vi "resources read.vi"(8 "error in":errorcluster, 10 "id":i32, 11 "message json":string) -> (0 "error out":errorcluster, 3 "response":string)   [LabVIEW 2025, in "MCP Server.lvlib"]
uses:
  MCP Server.lvlib
  53053a3e-d98d-4b1b-9ea2-8aa51a7e4ea3.vi
  26a76da7-6ace-4620-8e47-f7e66d57a6fb.vi
  a3b2ea05-9a55-4a6d-83fc-f98ed783a032.vi
  e0fbd291-d89e-42a3-8ed1-33df253c9476.vi
  fa2b7325-da3b-4faf-97be-a89ba966e5b3.vi
  <vilib>/JDP Science/JSONtext/Find Item.vi
  <vilib>/JDP Science/JSONtext/Next JSON Value.vi
  <vilib>/JDP Science/JSONtext/String Subset.vi
  <vilib>/JDP Science/JSONtext/Parsing/Advance past next JSON Value (inlined COPY).vi
  <vilib>/JDP Science/JSONtext/Parsing/Advance past whitespace.vi
  <vilib>/JDP Science/JSONtext/Parsing/Advance past String.vi
  <vilib>/JDP Science/JSONtext/Parsing/Advance past Number.vi
  <vilib>/JDP Science/JSONtext/Parsing/Advance past Line Ending.vi
  <vilib>/JDP Science/JSONtext/Parsing/Parse Full Path or Item Name.vi
  <vilib>/JDP Science/JSONtext/Parsing/Advance past Array.vi
  <vilib>/JDP Science/JSONtext/Parsing/Advance past Object.vi
  <vilib>/JDP Science/JSONtext/support/Error Cluster From Code.vi
  <vilib>/JDP Science/JSONtext/Offset/Find Item Locations by Path.vi
  <vilib>/JDP Science/JSONtext/JSON text to Variant.vi
  <vilib>/Utility/error.llb/Error Cluster From Error Code.vi
  <vilib>/JDP Science/JSONtext/Variant to JSON Text.vi
  <vilib>/JDP Science/JSONtext/support/Format JSON Array Text.vi
  <vilib>/JDP Science/JSONtext/support/Format JSON Object.vi
  <vilib>/JDP Science/JSONtext/LVClass Serializer/JSONtext LVClass Serializer.lvclass
  <vilib>/ErrorRing/Error Ring.xnode
  <vilib>/JDP Science/JSONtext/JSONtext.lvlib
  <vilib>/JDP Science/JDP Science Common Utilities/Base64/Base64 Support.lvlib
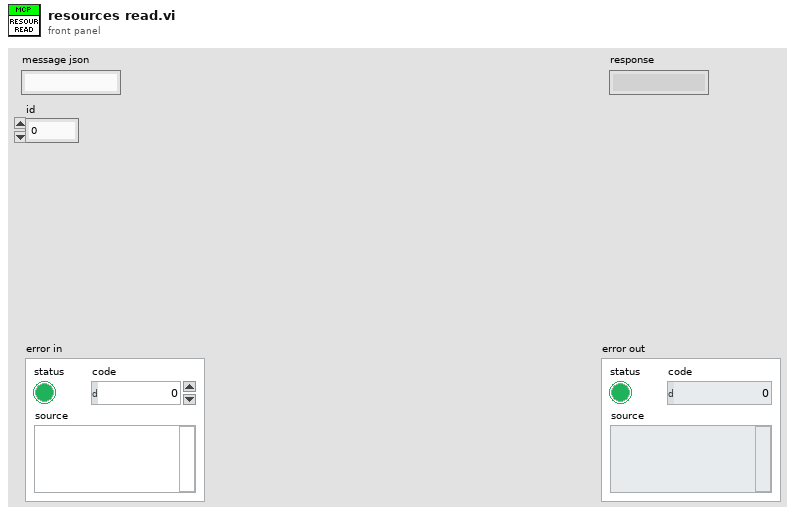
[diagram p1: front panel]
types:
  T1 = typedef "MCP Server.lvlib/resource data.ctl" = cluster{"uri":string, "name":string, "description":string, "mimeType":string, "file path":path}
  T2 = cluster{"uri":string, "mimeType":string, "text":string}
  T3 = cluster{"uri":string, "mimeType":string, "blob":string}
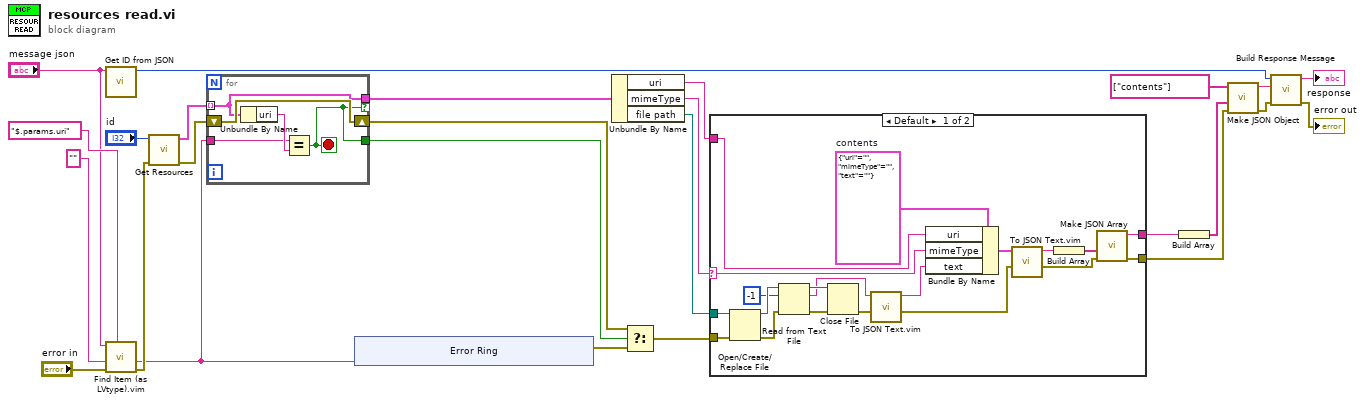
[diagram p0: block diagram]
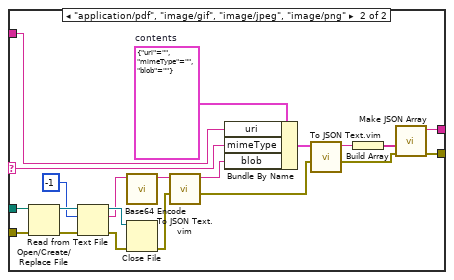
[diagram p2: hidden frame]
diagram:
  n1 = call "Get ID from JSON.vi"("message json"="message json") -> ("Data out"=w8:i32)  [unwired: 10 in]
  n2 = call "Find Item (as LVtype).vim"("$Path or Item Name"="$.params.uri", "error in (no error)"="error in", "Data Type and Default Value"="" ("JSON"), "JSON"="message json") -> ("error out"=w21:errorcluster, "Data"=w12:string)  [unwired: 4 in, 2 out]
  n3 = call "Get Resources.vi"("error in (no error)"=w21, "id"="id") -> ("error out"=w25:errorcluster, "resources"=w22:T1[])  [unwired: 8 in]
  n4 = for {
    shift-right: [w31] -> w23
    shift-left: w25 -> [w31]
    tunnel: w22 -> [w28] mode=indexing
    tunnel: w12 -> [w29]
    tunnel: [w28] -> w18 if=w27
    tunnel: [w27] -> w15
    stop <- w27 stop-if-true
    n5 = Unbundle By Name(w28) -> ("uri"=w30:string)
    n6 = Equal?(x=w29, y=w30) -> (x = y?=w27:bool)
  }
  n7 = xnode "Error Ring"("parameter 0"=w12) -> ("error out"=w16:errorcluster)
  n8 = Unbundle By Name(w18) -> ("uri"=w7:string, "mimeType"=w13:string, "file path"=w6:path)
  n9 = Select(t=w23, s=w15, f=w16) -> (s? t:f=w17:errorcluster)
  n10 = case shown="Default" w13 {
    selector: w13 -> [w44 w65]
    tunnel: w17 -> [w51 w72]
    tunnel: [w37 w59] -> w14
    tunnel: w7 -> [w43 w64]
    tunnel: [w36 w58] -> w3
    tunnel: w6 -> [w33 w55]
    frame Default {
      w45 = T2 {"uri"="", "mimeType"="", "text"=""}  # contents
      n11 = Open/Create/Replace File(file path (use dialog)=w33, error in=w51) -> (refnum out=w47:refnum<file>, error out=w50:errorcluster)  [unwired: 4 in, 1 out]
      n12 = Read from Text File(file (use dialog)=w47, count=-1, error in=w50) -> (refnum out=w46:refnum<file>, text=w41:string, error out=w49:errorcluster)  [unwired: 1 in, 1 out]
      n13 = Close File(refnum=w46, error in=w49) -> (error out=w48:errorcluster)  [unwired: 1 out]
      n14 = call "To JSON Text.vim"("error in (no error)"=w48, "Anything"=w41) -> ("error out"=w42:errorcluster, "<JSON>"=w40:string)  [unwired: 8 in]
      n15 = Bundle By Name(cluster=w45, "uri"=w43, "mimeType"=w44, "text"=w40) -> (w38:T2)
      n16 = call "To JSON Text.vim"("error in (no error)"=w42, "Anything"=w38) -> ("error out"=w39:errorcluster, "<JSON>"=w35:string)  [unwired: 8 in]
      n17 = Build Array(w35) -> (w34:string[])
      n18 = call <vilib>:"Make JSON Array.vi"("error in (no error)"=w39, "JSON Elements"=w34) -> ("error out"=w37:errorcluster, "<JSON>"=w36:string)  [unwired: 8 in]
    }
    frame "application/pdf", "image/gif", "image/jpeg", "image/png" {
      w66 = T3 {"uri"="", "mimeType"="", "blob"=""}  # contents
      n19 = Open/Create/Replace File(file path (use dialog)=w55, error in=w72) -> (refnum out=w68:refnum<file>, error out=w71:errorcluster)  [unwired: 4 in, 1 out]
      n20 = Read from Text File(file (use dialog)=w68, count=-1, error in=w71) -> (refnum out=w67:refnum<file>, text=w53:string, error out=w70:errorcluster)  [unwired: 1 in, 1 out]
      n21 = call <vilib>:"Base64 Encode.vi"("String to Encode"=w53) -> ("Base64 Encoded"=w52:string)  [unwired: 10 in]
      n22 = Close File(refnum=w67, error in=w70) -> (error out=w69:errorcluster)  [unwired: 1 out]
      n23 = call "To JSON Text.vim"("error in (no error)"=w69, "Anything"=w52) -> ("error out"=w63:errorcluster, "<JSON>"=w62:string)  [unwired: 8 in]
      n24 = Bundle By Name(cluster=w66, "uri"=w64, "mimeType"=w65, "blob"=w62) -> (w60:T3)
      n25 = call "To JSON Text.vim"("error in (no error)"=w63, "Anything"=w60) -> ("error out"=w61:errorcluster, "<JSON>"=w57:string)  [unwired: 8 in]
      n26 = Build Array(w57) -> (w56:string[])
      n27 = call <vilib>:"Make JSON Array.vi"("error in (no error)"=w61, "JSON Elements"=w56) -> ("error out"=w59:errorcluster, "<JSON>"=w58:string)  [unwired: 8 in]
    }
  }
  n28 = Build Array(w3) -> (w2:string[])
  n29 = call <vilib>:"Make JSON Object.vi"("error in (no error)"=w14, "JSON Items"=w2, "Item Names"=string[] ["contents"]) -> ("error out"=w5:errorcluster, "<JSON>"=w1:string)  [unwired: 7 in]
  n30 = call "Build Response Message.vi"("error in (no error)"=w5, "Result content"=w1, "message id in"=w8) -> ("error out"=→"error out":errorcluster, "MCP message out"=→"response":string)  [unwired: 7 in]
